vi "xml generate for SFP+_VNA.vi"(0 "input_array_SDD11_Max":string[](array[string]), 1 "input_array_SDD21":string[](array[string]), 2 "路径":path=path "D:/wmgxml.xml", 3 "input_str_label":string, 4 "input_str_CustomerPN":string, 5 "input_array_SCC11_Max":string[](array[string]), 6 "FilePath":string, 7 "input_array_ILD_Max":string[](array[string]), 8 "FileVer":string, 9 "input_array_TDD11":string[](array[string]), 11 "input_array_TDD22":string[](array[string]), 12 "input_array_Next":string[](array[string]), 13 "input_array_time":string[](array[string]), 14 "input_array_impSpec":string[](array[string])) -> ()   [LabVIEW 2011]
panel:
  out "TDD":string
  out "NEXT":string
  out "SCC11":string
  out "SCD21-SDD21":string
  out "ILD":string
  out "SDD11":string
  out "SDD21":string
  in  "input_test_results":bool[](array[boolean])
  out "midVar_time":string[](array[string])
  in  "midVar_state":string
  in  "input_str_product":string
  out "midVar_Content":string
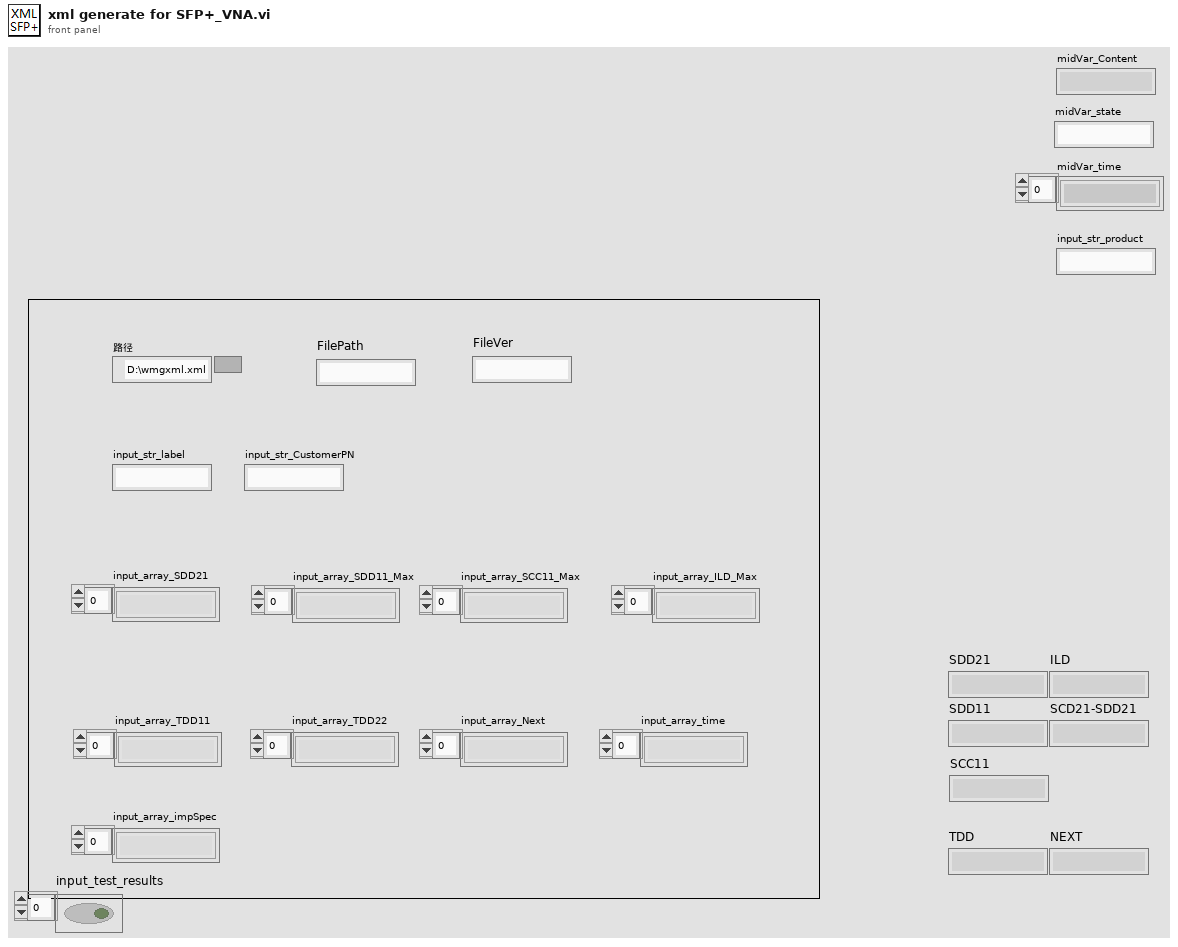
[diagram p1: front panel]
types:
  T1 = enum16{"open", "replace", "create", "open or create", "replace or create", "replace or create with confirmation"}
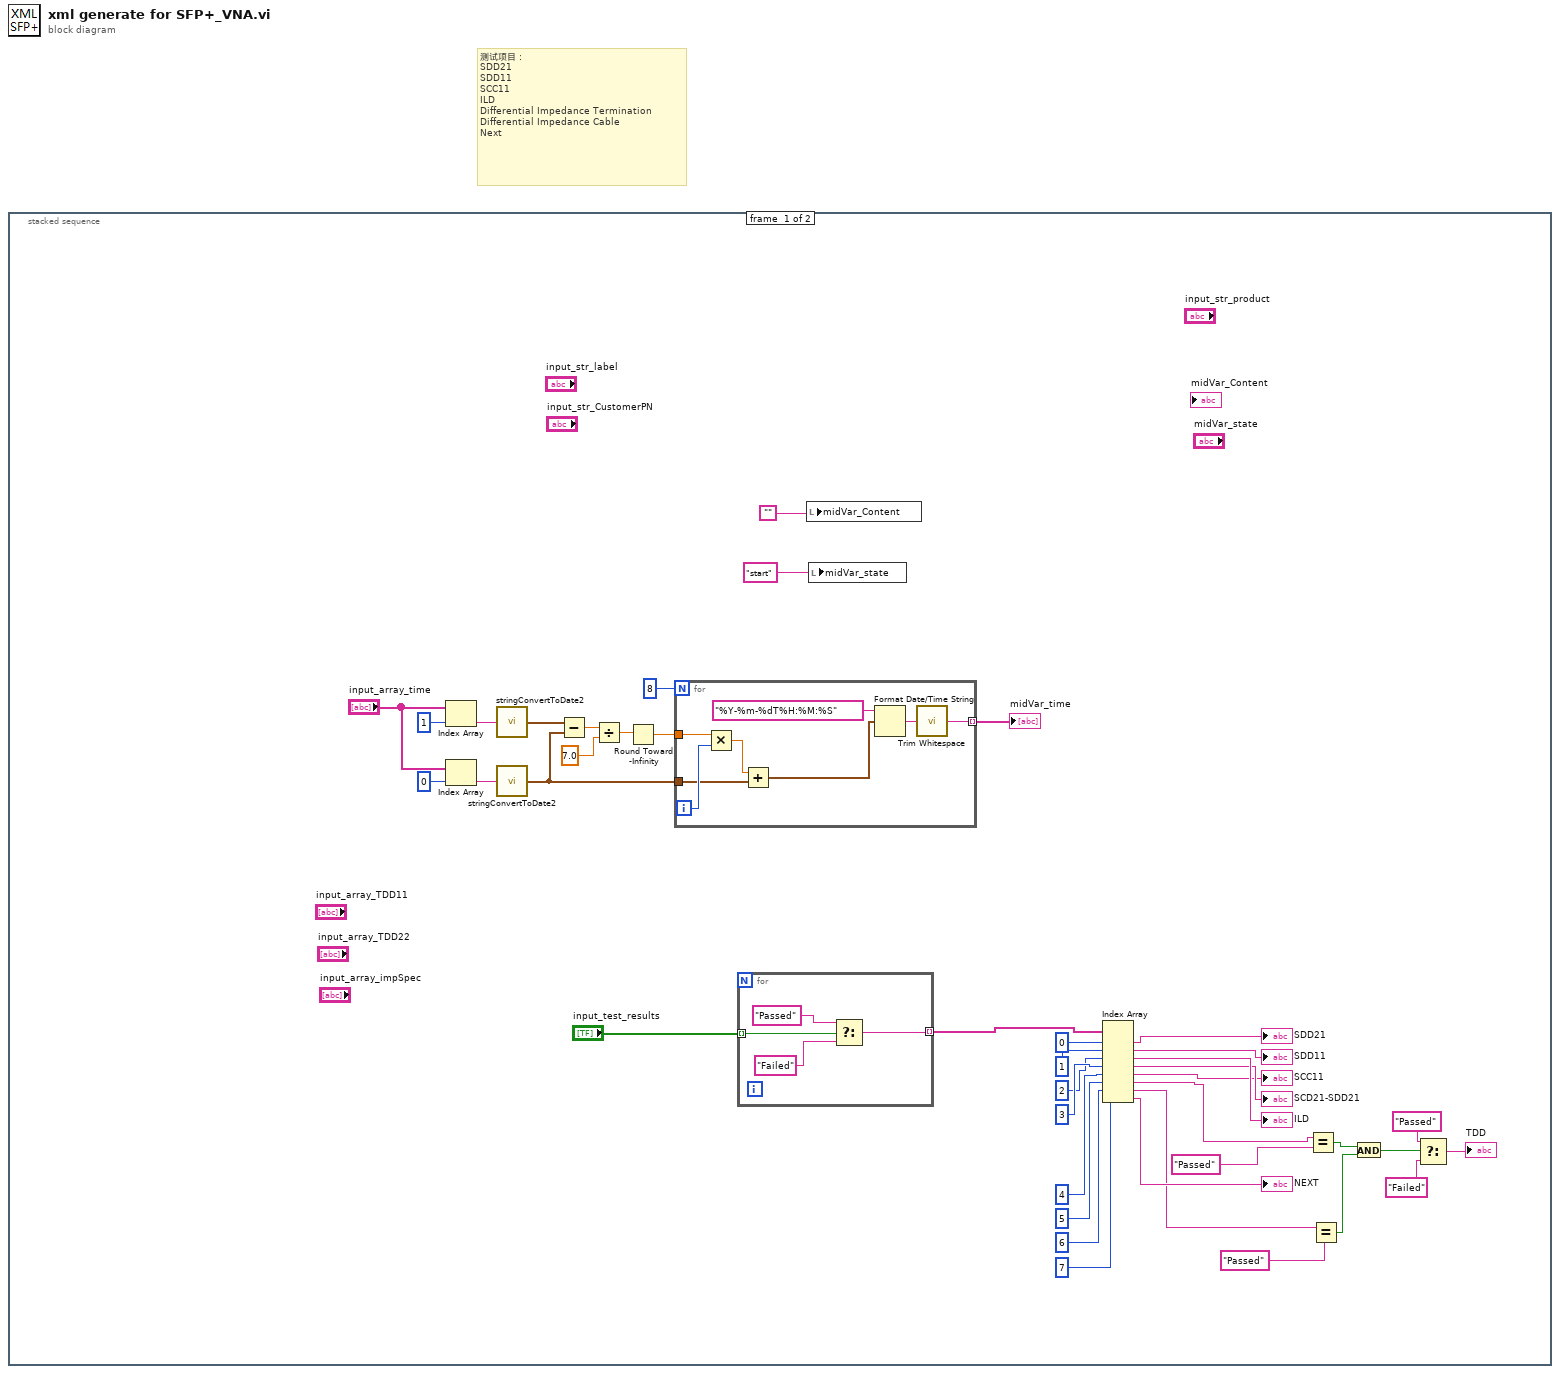
[diagram p0: block diagram]
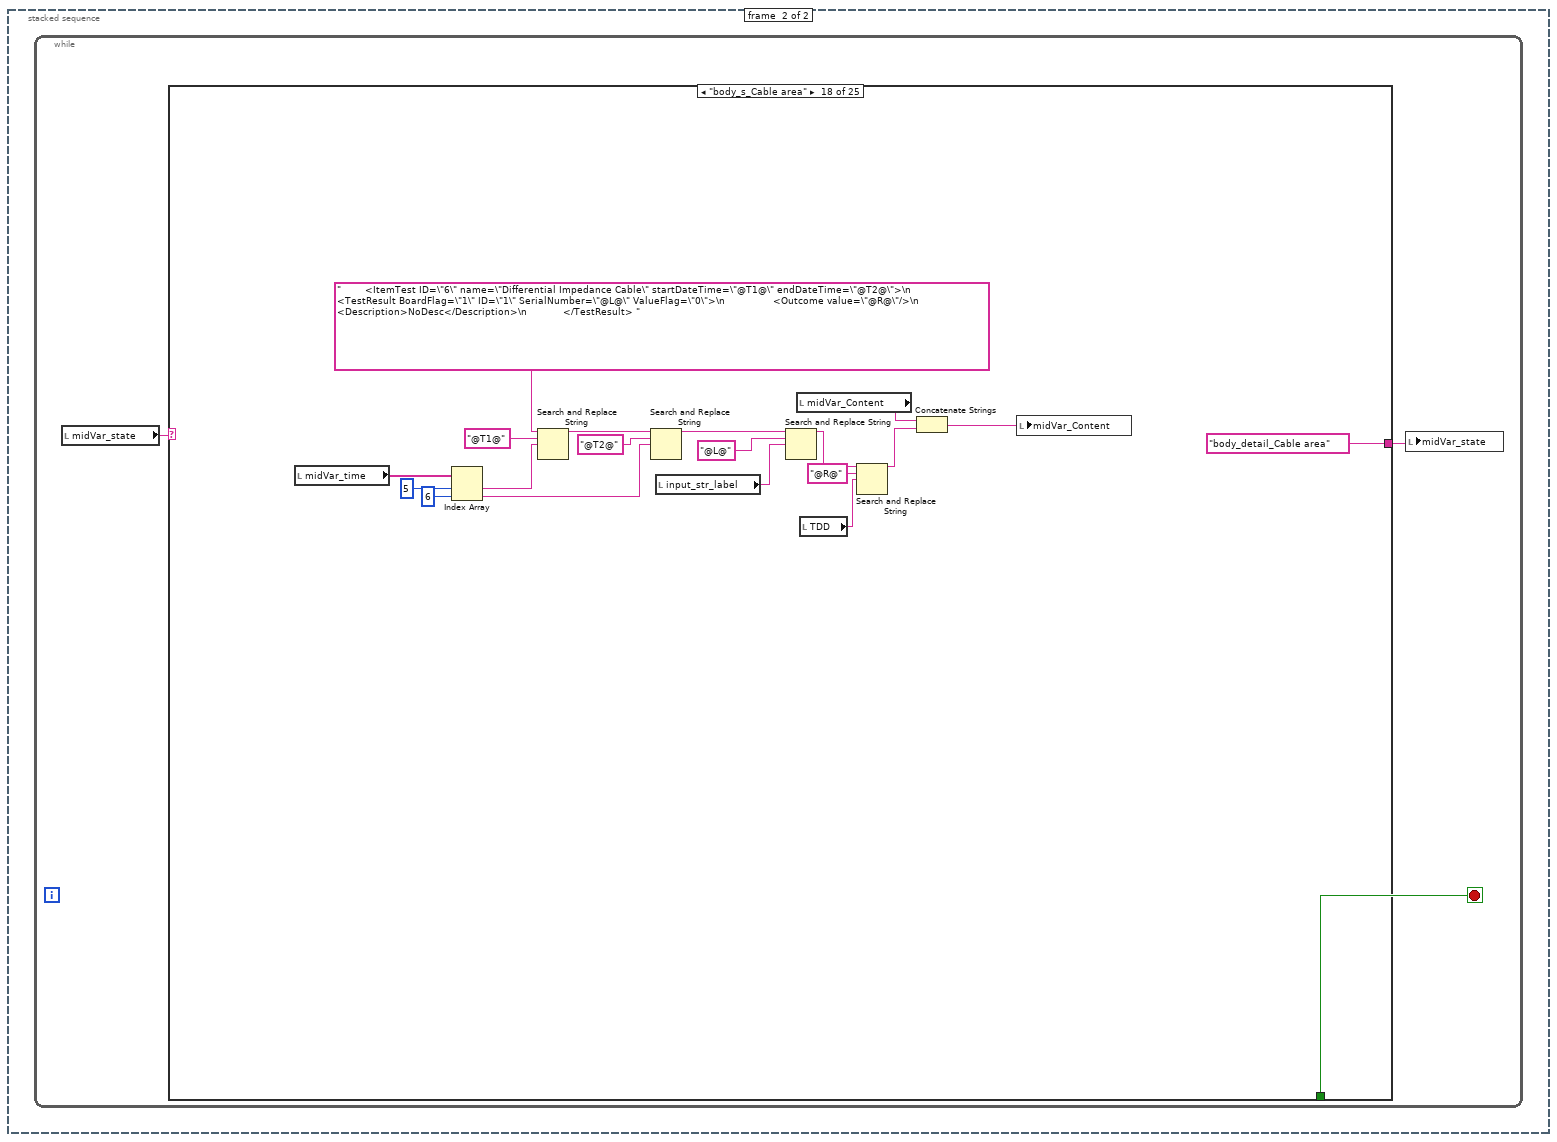
[diagram p2: hidden frame]
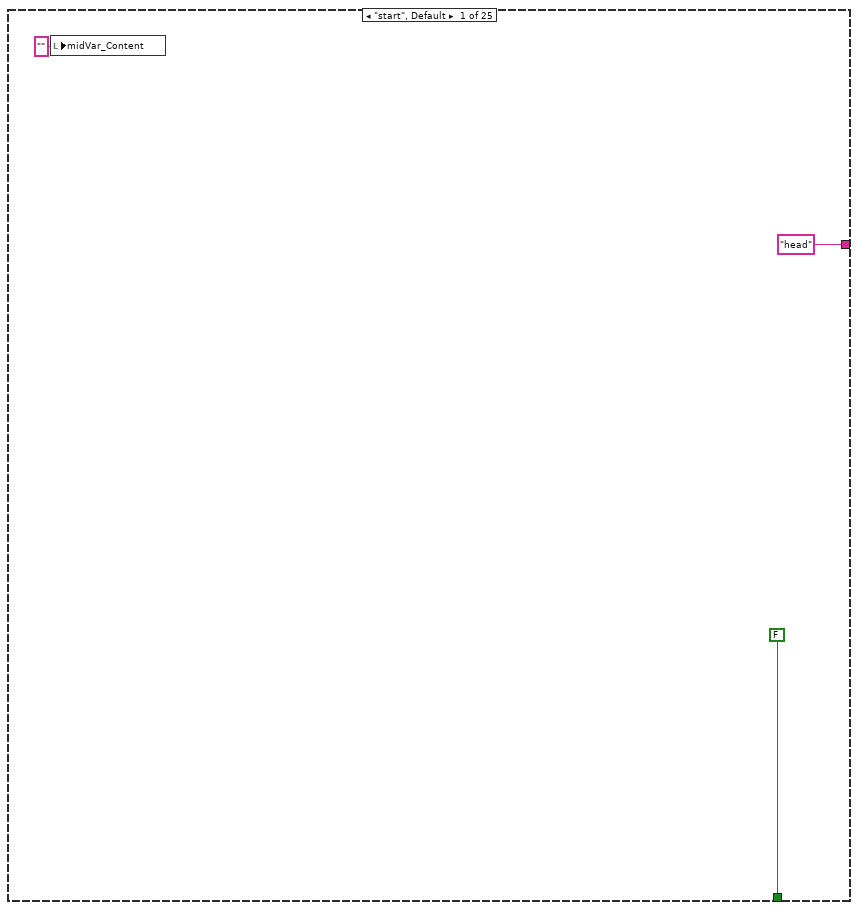
[diagram p3: hidden frame]
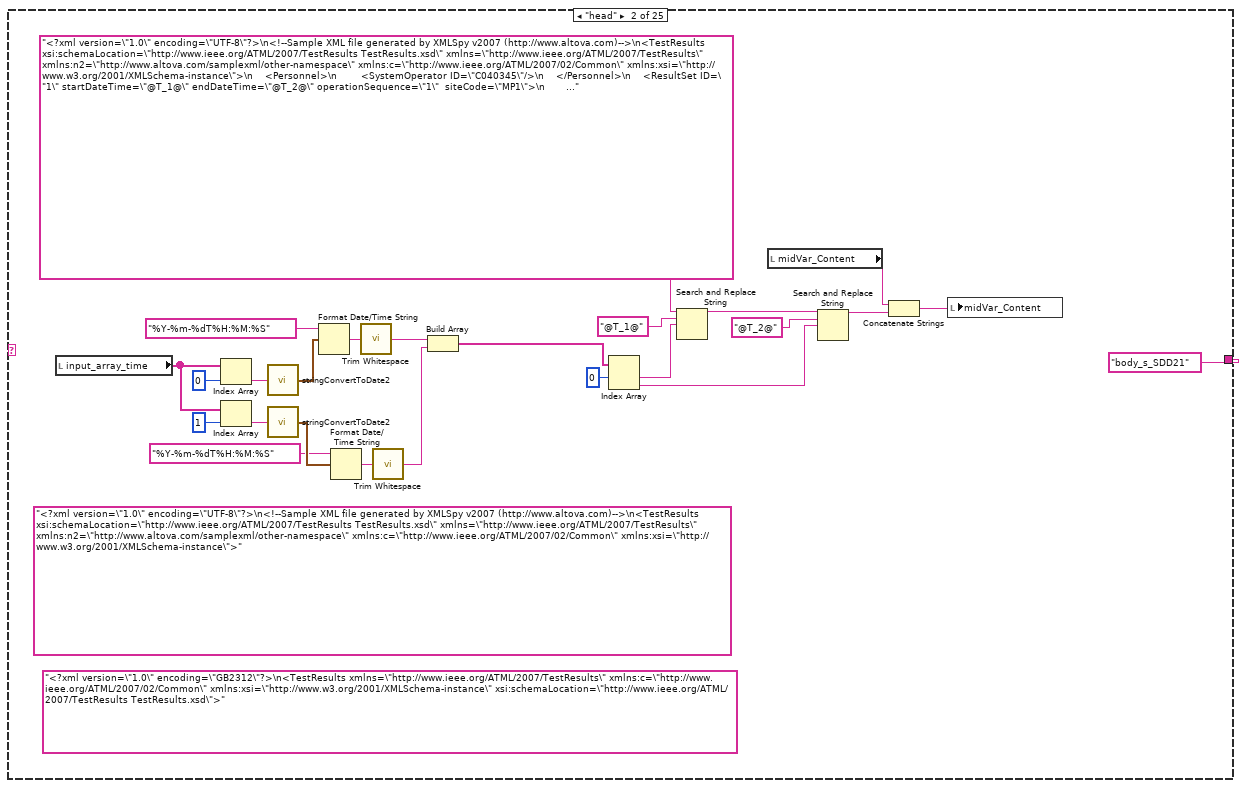
[diagram p4: hidden frame]
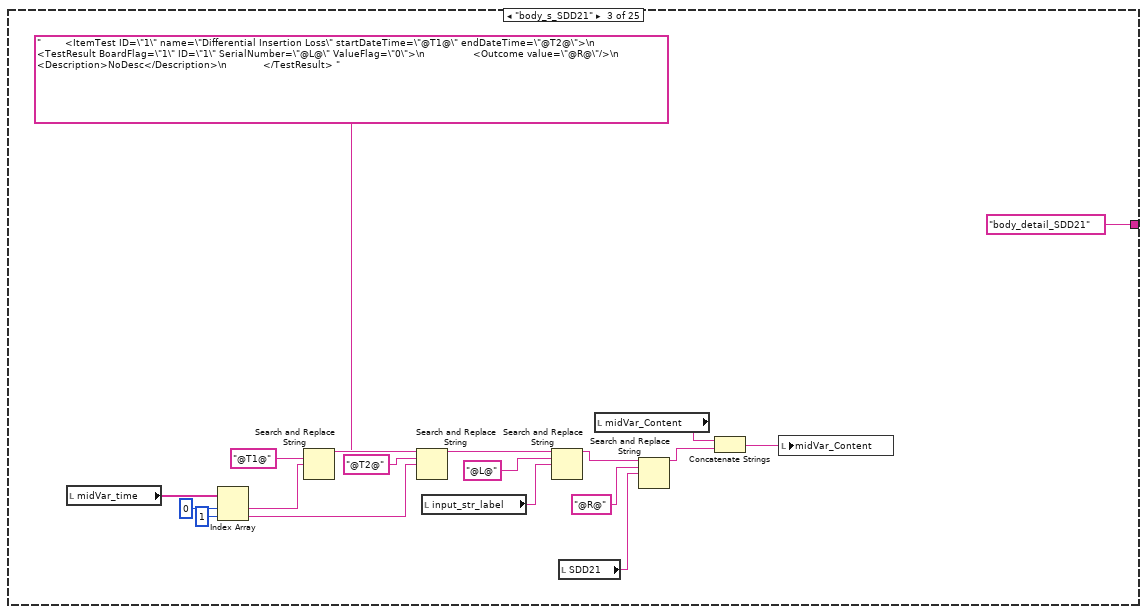
[diagram p5: hidden frame]
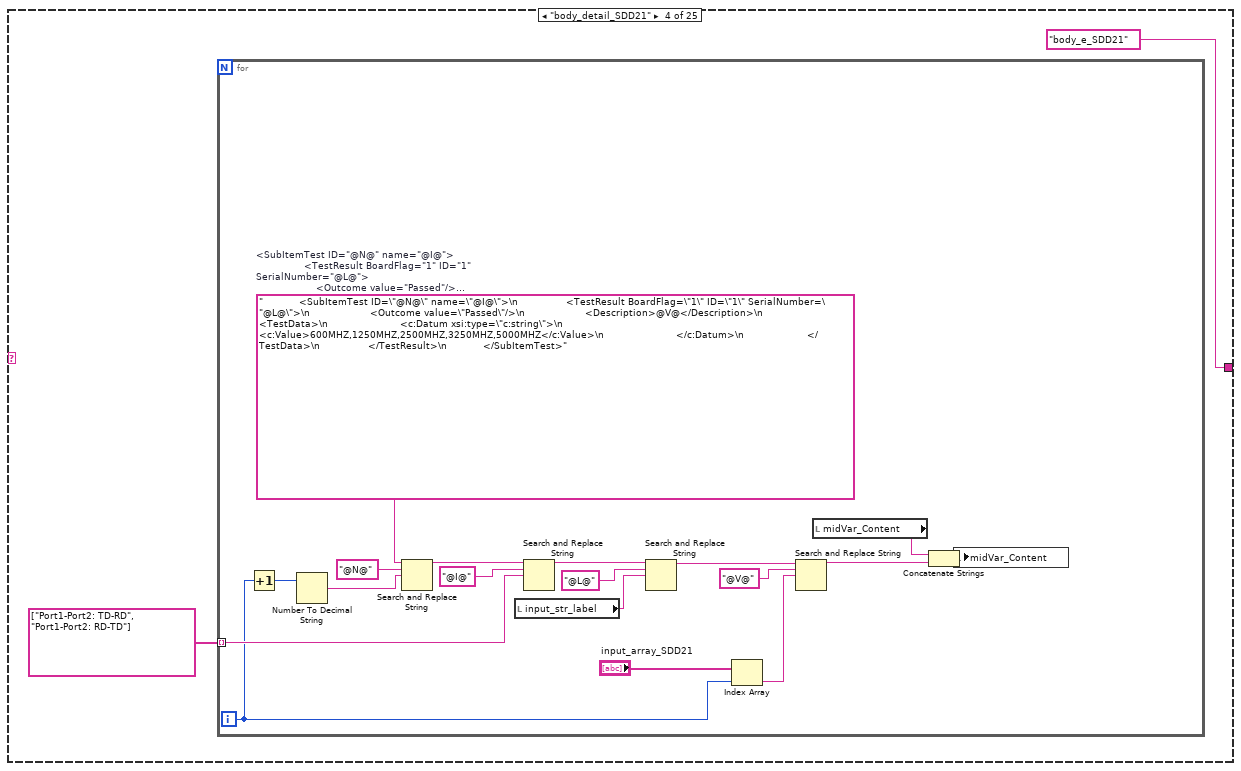
[diagram p6: hidden frame]
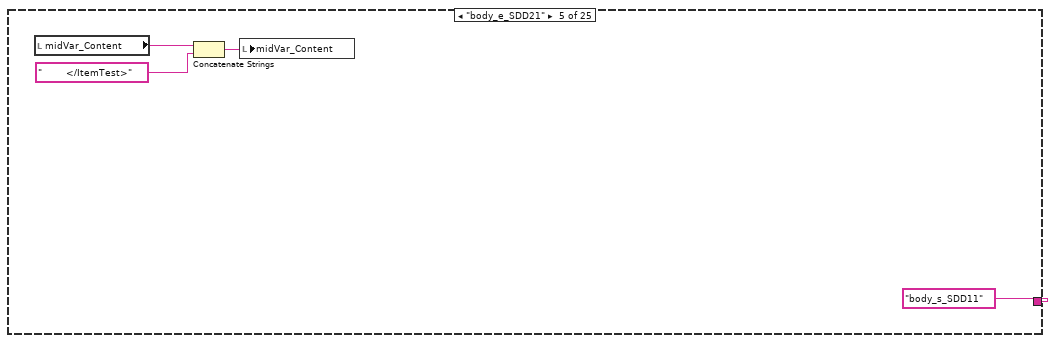
[diagram p7: hidden frame]
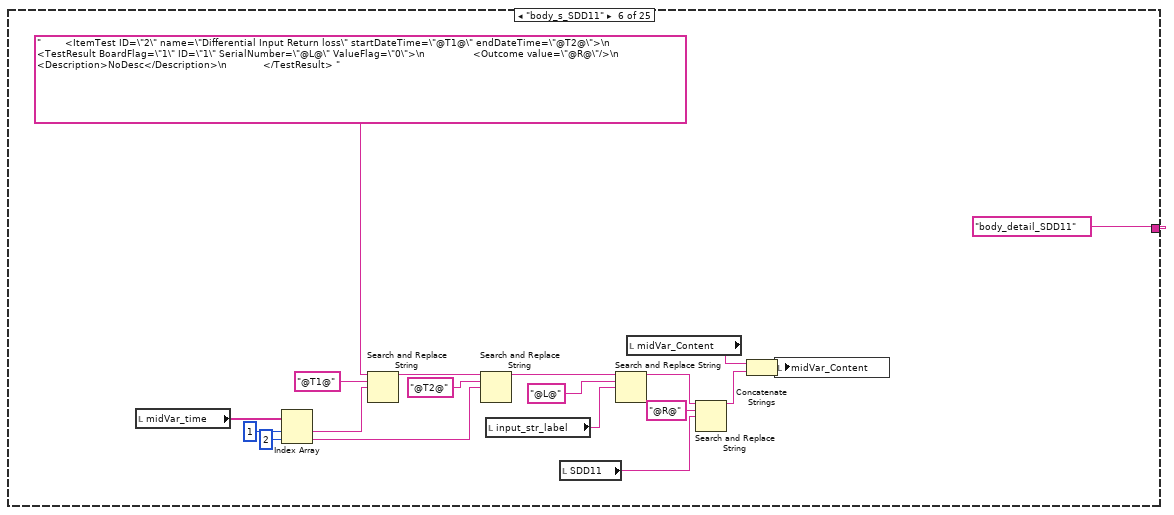
[diagram p8: hidden frame]
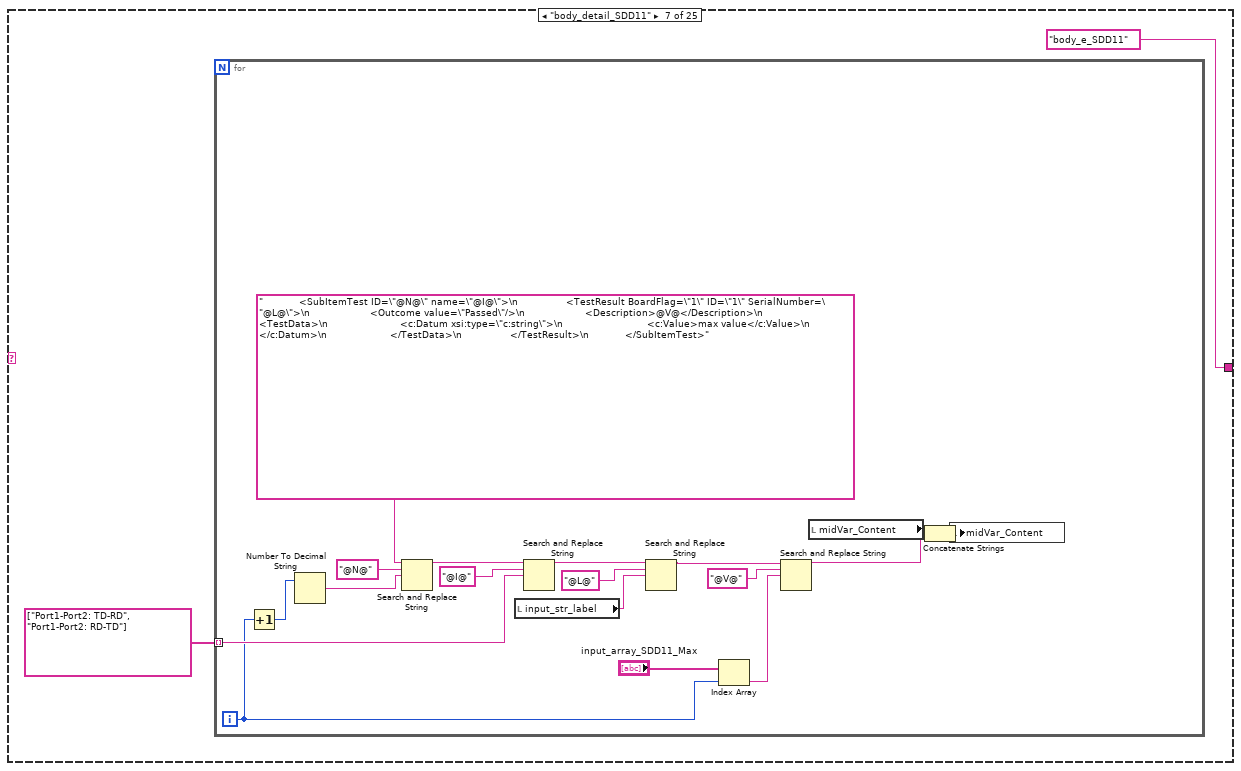
[diagram p9: hidden frame]
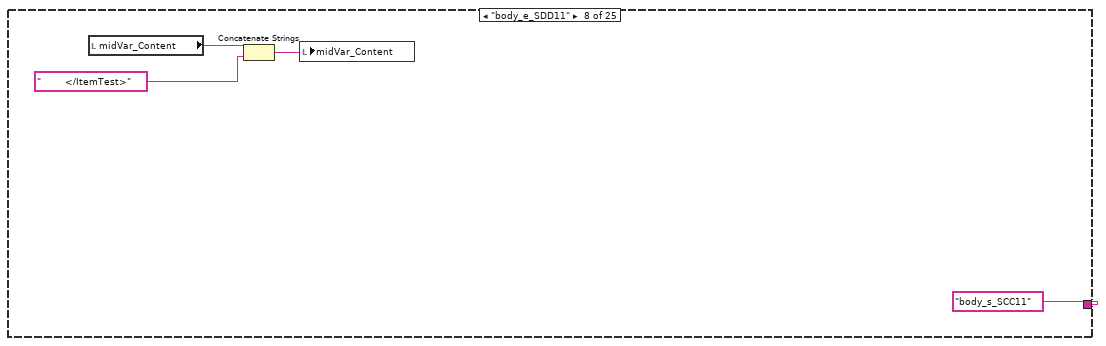
[diagram p10: hidden frame]
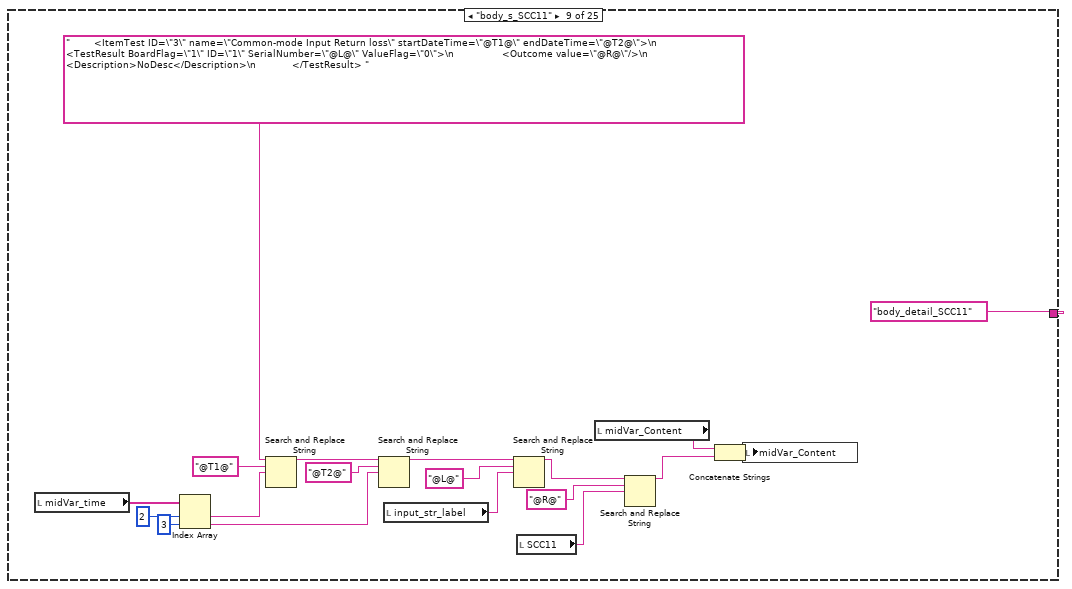
[diagram p11: hidden frame]
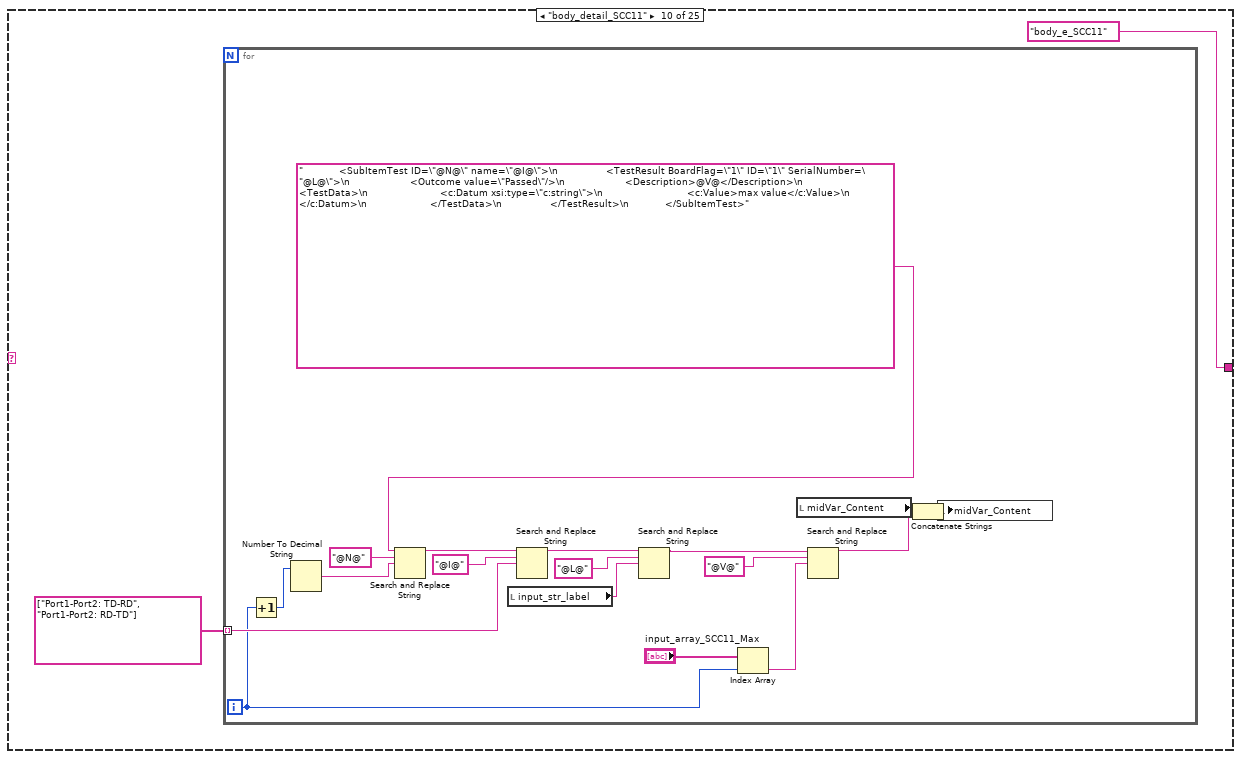
[diagram p12: hidden frame]
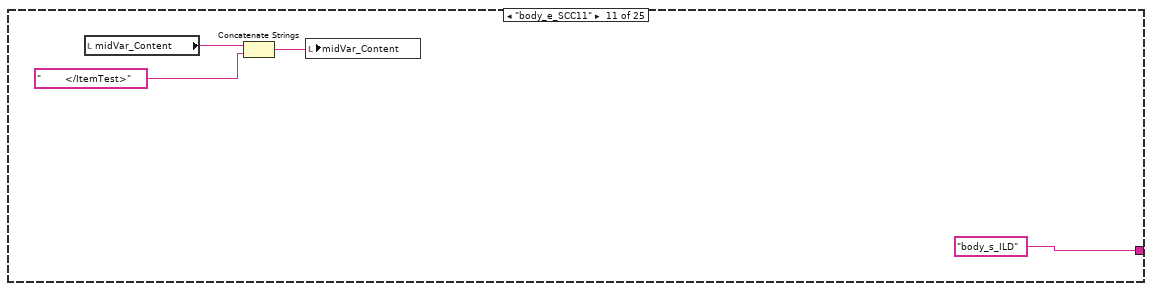
[diagram p13: hidden frame]
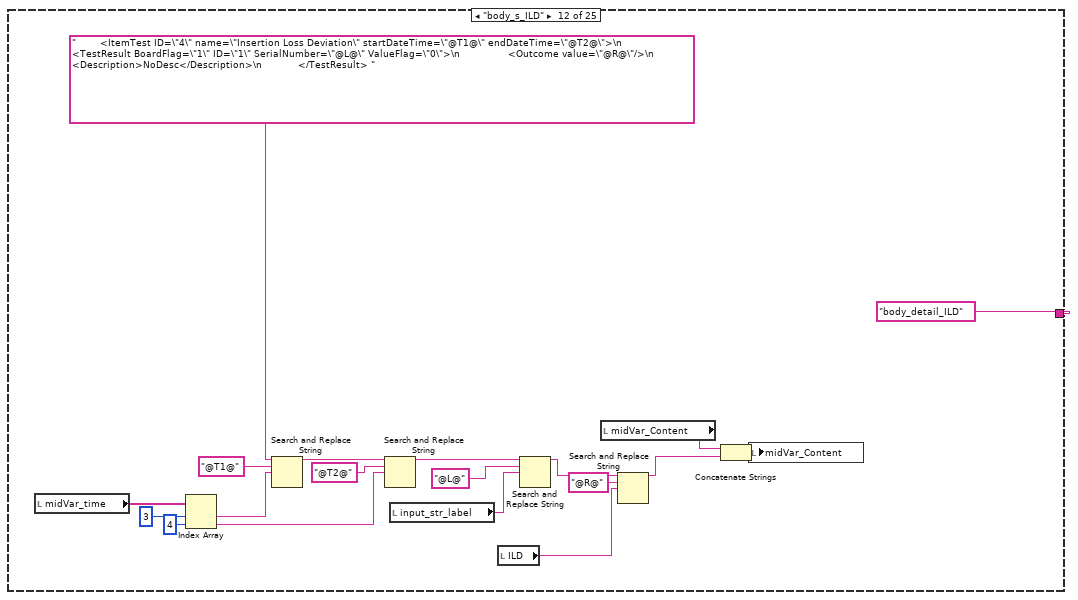
[diagram p14: hidden frame]
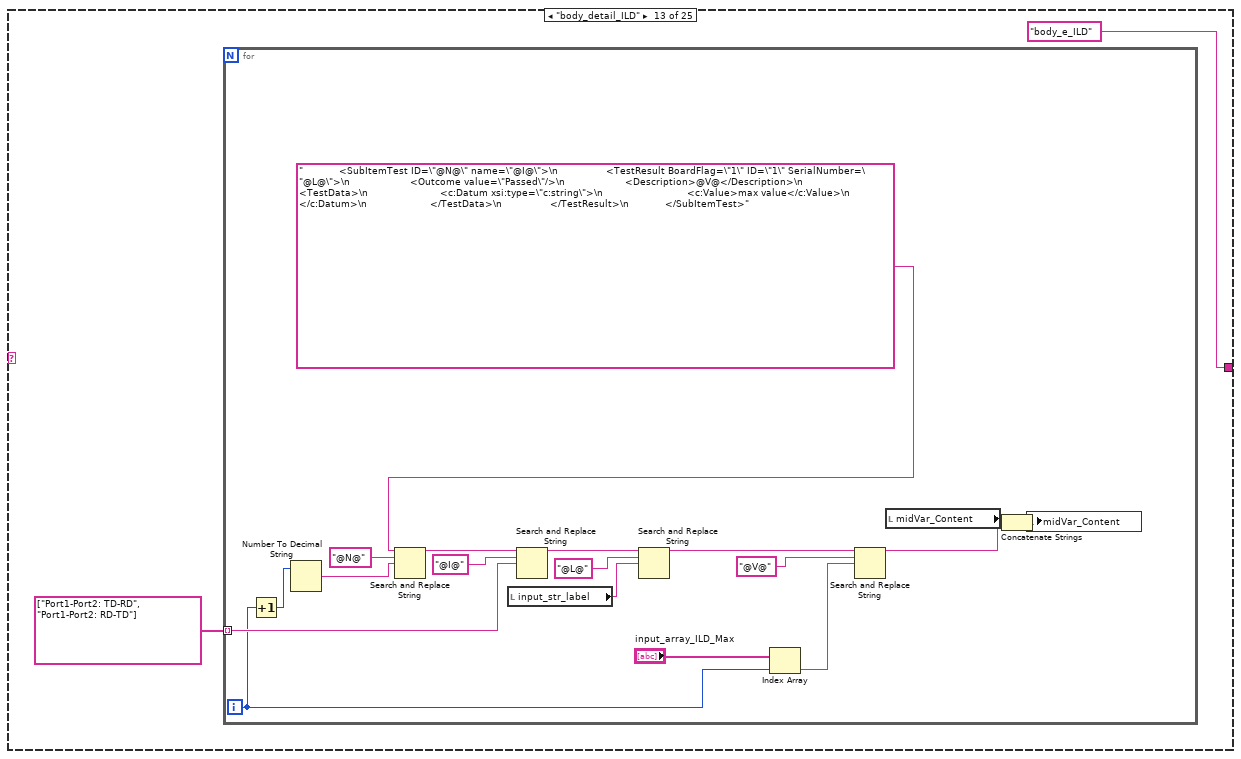
[diagram p15: hidden frame]
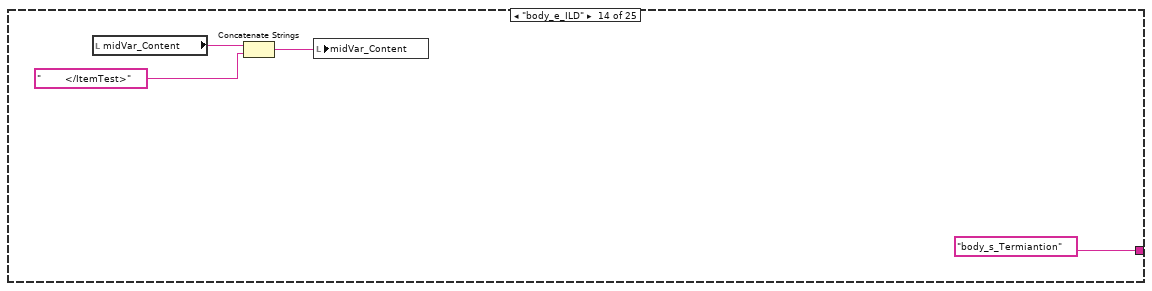
[diagram p16: hidden frame]
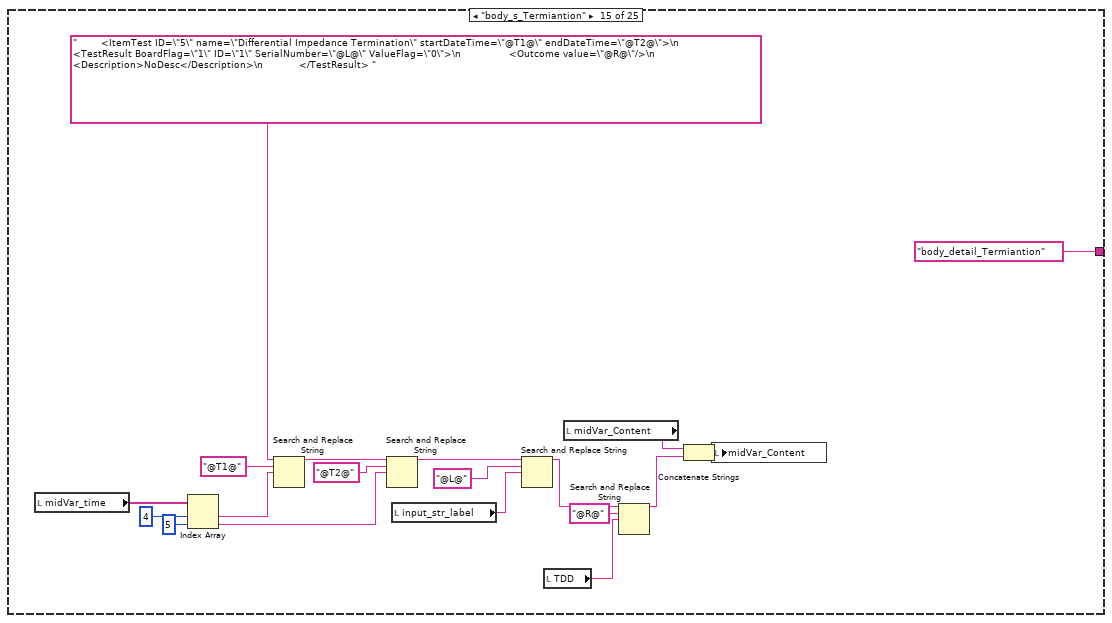
[diagram p17: hidden frame]
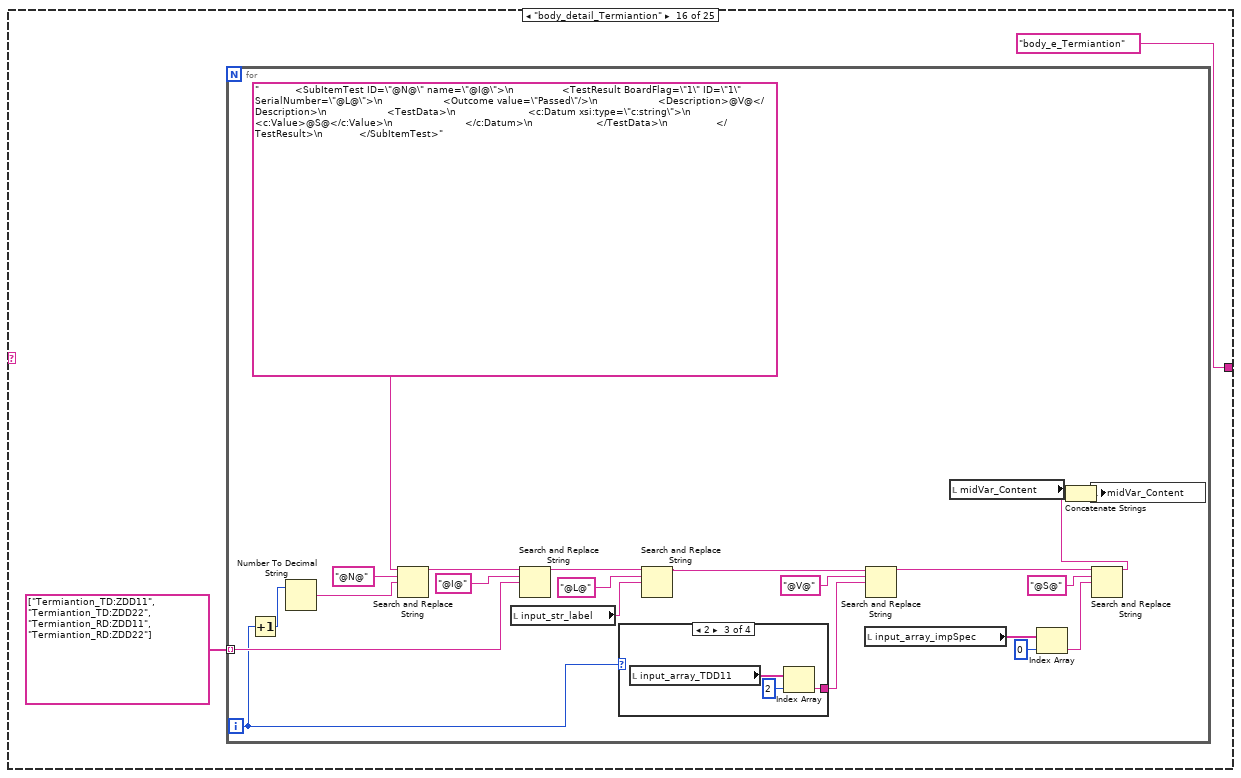
[diagram p18: hidden frame]
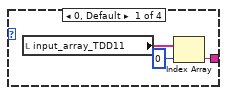
[diagram p19: hidden frame]
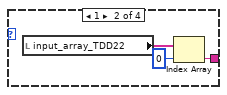
[diagram p20: hidden frame]
diagram:
  # "测试项目：\nSDD21\nSDD11\nSCC11\nILD\nDifferential Impedance Termination\nDifferential Impedance Cable\nNext"
  n1 = stacked-sequence {
    frame #0 {
      n2 = Index Array(array="input_array_time", index=1 ("索引")) -> (element=w30:string)
      n3 = Index Array(array="input_array_time", index=0 ("索引")) -> (element=w31:string)
      n4 = call "stringConvertToDate2.vi"("input_str_yymmdd"=w30) -> ("show_date"=w32:timestamp)
      n5 = call "stringConvertToDate2.vi"("input_str_yymmdd"=w31) -> ("show_date"=w38:timestamp)
      n6 = Subtract(x=w32, y=w38) -> (x-y=w33:dbl)
      n7 = Divide(x=w33, y=7.0) -> (x/y=w35:dbl)
      n8 = Round Toward -Infinity(1:w35) -> (0:w37:dbl)
      n9 = for {
        N: 8 -> [_]
        tunnel: w37 -> [w53]
        tunnel: w38 -> [w51]
        tunnel: [w46] -> w39 mode=indexing
        i -> [w52]
        n10 = Multiply(x=w53, y=w52) -> (x*y=w50:dbl)
        n11 = Add(x=w50, y=w51) -> (x+y=w47:timestamp)
        n12 = Format Date/Time String(time format string (%c)="%Y-%m-%dT%H:%M:%S" ("时间格式字符串(%c)"), seconds (now)=w47) -> (date/time string=w48:string)  [unwired: 1 in]
        n13 = call <vilib>:"Trim Whitespace.vi"("string"=w48) -> ("trimmed string"=w46:string)  [unwired: 1 in]
      }
      "midVar_time" <- w39
      n14 = for {
        tunnel: "input_test_results" -> [w45] mode=indexing
        tunnel: [w42] -> w25 mode=indexing
        n15 = Select(t="Passed", s=w45, f="Failed") -> (s? t:f=w42:string)
      }
      n16 = local write "midVar_Content"("") -> ()
      n17 = local write "midVar_state"("start" ("state")) -> ()
      n18 = Index Array(array=w25, index #1=0 ("索引"), index #2=1 ("索引"), index #3=2 ("索引"), index #4=3 ("索引"), index #5=4 ("索引"), index #6=5 ("索引"), index #7=6 ("索引"), index #8=7 ("索引")) -> (element #1=→"SDD21":string, element #2=→"SDD11":string, element #3=→"ILD":string, element #4=→"SCD21-SDD21":string, element #5=→"SCC11":string, element #6=w11:string, element #7=w9:string, element #8=→"NEXT":string)
      n19 = Equal?(x=w11, y="Passed") -> (x = y?=w7:bool)
      n20 = Equal?(x=w9, y="Passed") -> (x = y?=w6:bool)
      n21 = And(x=w7, y=w6) -> (x .and. y?=w5:bool)
      n22 = Select(t="Passed", s=w5, f="Failed") -> (s? t:f=→"TDD":string)
    }
    frame #1 {
      n23 = while {
        stop <- w54 stop-if-true
        n24 = local read "midVar_state"() -> (w56:string)
        n25 = case shown="\"body_s_Cable area\"" w56 {
          tunnel: ["head" ("state") "body_s_SDD21" ("state") "body_detail_SDD21" "body_e_SDD21" "body_s_SDD11" "body_detail_SDD11" "body_e_SDD11" "body_s_SCC11" "body_detail_SCC11" "body_e_SCC11" "body_s_ILD" "body_detail_ILD" "body_e_ILD" "body_s_Termiantion" "body_detail_Termiantion" "body_e_Termiantion" "body_s_Cable area" "body_detail_Cable area" "body_e_Cable area" "body_s_Next" "body_detail_Next" "body_e_Next" "tail" "end" ("state") "start" ("state")] -> w55
          tunnel: [FALSE _ _ _ _ _ _ _ _ _ _ _ _ _ _ _ _ _ _ _ _ _ _ _ TRUE] -> w54
          frame "start", Default {
            n26 = local write "midVar_Content"("" ("字符串")) -> ()
          }
          frame "head" {
            (unwired) "<?xml version=\"1.0\" encoding=\"GB2312\"?>\n<TestResults xmlns=\"http://www.ieee.org/ATML/2007/TestResults\" xmlns:c=\"http://www.ieee.org/ATML/2007/02/Common\" xmlns:xsi=\"http://www.w3.org/2001/XMLSchema-instance\" xsi:schemaLocation=\"http://www.ieee.org/ATML/2007/TestResults TestResults.xsd\">"
            (unwired) "<?xml version=\"1.0\" encoding=\"UTF-8\"?>\n<!--Sample XML file generated by XMLSpy v2007 (http://www.altova.com)-->\n<TestResults xsi:schemaLocation=\"http://www.ieee.org/ATML/2007/TestResults TestResults.xsd\" xmlns=\"http://www.ieee.org/ATML/2007/TestResults\" xmlns:n2=\"http://www.altova.com/samplexml/other-namespace\" xmlns:c=\"http://www.ieee.org/ATML/2007/02/Common\" xmlns:xsi=\"http://www.w3.org/2001/XMLSchema-instance\">"
            n27 = local read "input_array_time"() -> (w69:string[])
            n28 = Index Array(array=w69, index=0 ("索引")) -> (element=w68:string)
            n29 = Index Array(array=w69, index=1 ("索引")) -> (element=w67:string)
            n30 = call "stringConvertToDate2.vi"("input_str_yymmdd"=w68) -> ("show_date"=w65:timestamp)
            n31 = call "stringConvertToDate2.vi"("input_str_yymmdd"=w67) -> ("show_date"=w64:timestamp)
            n32 = Format Date/Time String(time format string (%c)="%Y-%m-%dT%H:%M:%S" ("时间格式字符串(%c)"), seconds (now)=w65) -> (date/time string=w72:string)  [unwired: 1 in]
            n33 = Format Date/Time String(time format string (%c)="%Y-%m-%dT%H:%M:%S" ("时间格式字符串(%c)"), seconds (now)=w64) -> (date/time string=w66:string)  [unwired: 1 in]
            n34 = call <vilib>:"Trim Whitespace.vi"("string"=w72) -> ("trimmed string"=w62:string)  [unwired: 1 in]
            n35 = call <vilib>:"Trim Whitespace.vi"("string"=w66) -> ("trimmed string"=w61:string)  [unwired: 1 in]
            n36 = Build Array(w62, w61) -> (w60:string[])
            n37 = Index Array(array=w60, index #1=0 ("索引")) -> (element #1=w82:string, element #2=w79:string)  [unwired: 1 in]
            n38 = Search and Replace String(input string="<?xml version=\"1.0\" encoding=\"UTF-8\"?>\n<!--Sample XML file generated by XMLSpy v2007 (http://www.altova.com)-->\n<TestResults xsi:schemaLocation=\"http://www.ieee.org/ATML/2007/TestResults TestResults.xsd\" xmlns=\"http://www.ieee.org/ATML/2007/TestResults\" xmlns:n2=\"http://www.altova.com/samplexml/other-namespace\" xmlns:c=\"http://www.ieee.org/ATML/2007/02/Common\" xmlns:xsi=\"http://www.w3.org/2001/XMLSchema-instance\">\n    <Personnel>\n        <SystemOperator ID=\"C040345\"/>\n    </Personnel>\n    <ResultSet ID=\"1\" startDateTime=\"@T_1@\" endDateTime=\"@T_2@\" operationSequence=\"1\"  siteCode=\"MP1\">\n        <Description>CMZ00A2R</Description>\n        <TestResult BoardFlag=\"1\" ID=\"1\">\n            <Outcome value=\"Passed\"/>\n        </TestResult>", search string="@T_1@" ("搜索字符串"), replace string=w82) -> (result string=w81:string)  [unwired: 5 in, 3 out]
            n39 = local read "midVar_Content"() -> (w77:string)
            n40 = Search and Replace String(input string=w81, search string="@T_2@" ("搜索字符串"), replace string=w79) -> (result string=w74:string)  [unwired: 5 in, 3 out]
            n41 = Concatenate Strings(w77, w74) -> (w76:string)
            n42 = local write "midVar_Content"(w76) -> ()
          }
          frame "body_s_SDD21" {
            n43 = local read "midVar_time"() -> (w90:string[])
            n44 = Index Array(array=w90, index #1=0 ("索引"), index #2=1 ("索引")) -> (element #1=w101:string, element #2=w98:string)
            n45 = Search and Replace String(input string="        <ItemTest ID=\"1\" name=\"Differential Insertion Loss\" startDateTime=\"@T1@\" endDateTime=\"@T2@\">\n            <TestResult BoardFlag=\"1\" ID=\"1\" SerialNumber=\"@L@\" ValueFlag=\"0\">\n                <Outcome value=\"@R@\"/>\n                <Description>NoDesc</Description>\n            </TestResult> ", search string="@T1@" ("搜索字符串"), replace string=w101) -> (result string=w100:string)  [unwired: 5 in, 3 out]
            n46 = Search and Replace String(input string=w100, search string="@T2@" ("搜索字符串"), replace string=w98) -> (result string=w93:string)  [unwired: 5 in, 3 out]
            n47 = local read "input_str_label"() -> (w92:string)
            n48 = Search and Replace String(input string=w93, search string="@L@" ("搜索字符串"), replace string=w92) -> (result string=w88:string)  [unwired: 5 in, 3 out]
            n49 = local read "SDD21"() -> (w85:string)
            n50 = local read "midVar_Content"() -> (w97:string)
            n51 = Search and Replace String(input string=w88, search string="@R@" ("搜索字符串"), replace string=w85) -> (result string=w87:string)  [unwired: 5 in, 3 out]
            n52 = Concatenate Strings(w97, w87) -> (w96:string)
            n53 = local write "midVar_Content"(w96) -> ()
          }
          frame "body_detail_SDD21" {
            n54 = for {
              tunnel: string[] ["Port1-Port2: TD-RD", "Port1-Port2: RD-TD"] -> [w118] mode=indexing
              i -> [w108]
              w123 = "            <SubItemTest ID=\"@N@\" name=\"@I@\">\n                <TestResult BoardFlag=\"1\" ID=\"1\" SerialNumber=\"@L@\">\n                    <Outcome value=\"Passed\"/>\n                    <Description>@V@</Description>\n                    <TestData>\n                        <c:Datum xsi:type=\"c:string\">\n                            <c:Value>600MHZ,1250MHZ,2500MHZ,3250MHZ,5000MHZ</c:Value>\n                        </c:Datum>\n                     </TestData>\n                </TestResult>\n            </SubItemTest>"  # <SubItemTest ID="@N@" name="@I@">                 <TestResult BoardFlag="1" ID="1" SerialNumber="@L@">                     <Outcome value="Passed"/>                     <Description>@V@</Description>                     <TestData>                         <c:Datum xsi:type="c:string">                             <c:Value>600MHZ,1250MHZ,2500MHZ,3250MHZ,5000MHZ</c:Value>                         </c:Datum>                      </TestData>                 </TestResult>             </SubItemTest>
              n55 = Increment(x=w108) -> (x+1=w110:i32)
              n56 = Number To Decimal String(number=w110) -> (decimal integer string=w121:string)  [unwired: 1 in]
              n57 = Search and Replace String(input string=w123, search string="@N@" ("搜索字符串"), replace string=w121) -> (result string=w120:string)  [unwired: 5 in, 3 out]
              n58 = local read "input_str_label"() -> (w115:string)
              n59 = Search and Replace String(input string=w120, search string="@I@" ("搜索字符串"), replace string=w118) -> (result string=w117:string)  [unwired: 5 in, 3 out]
              n60 = Search and Replace String(input string=w117, search string="@L@" ("搜索字符串"), replace string=w115) -> (result string=w109:string)  [unwired: 5 in, 3 out]
              n61 = Index Array(array="input_array_SDD21", index=w108) -> (element=w112:string)
              n62 = Search and Replace String(input string=w109, search string="@V@" ("搜索字符串"), replace string=w112) -> (result string=w106:string)  [unwired: 5 in, 3 out]
              n63 = local read "midVar_Content"() -> (w114:string)
              n64 = Concatenate Strings(w114, w106) -> (w111:string)
              n65 = local write "midVar_Content"(w111) -> ()
            }
          }
          frame "body_e_SDD21" {
            n66 = local read "midVar_Content"() -> (w127:string)
            n67 = Concatenate Strings(w127, "        </ItemTest>") -> (w126:string)
            n68 = local write "midVar_Content"(w126) -> ()
          }
          frame "body_s_SDD11" {
            n69 = local read "midVar_time"() -> (w133:string[])
            n70 = Index Array(array=w133, index #1=1 ("索引"), index #2=2 ("索引")) -> (element #1=w144:string, element #2=w141:string)
            n71 = Search and Replace String(input string="        <ItemTest ID=\"2\" name=\"Differential Input Return loss\" startDateTime=\"@T1@\" endDateTime=\"@T2@\">\n            <TestResult BoardFlag=\"1\" ID=\"1\" SerialNumber=\"@L@\" ValueFlag=\"0\">\n                <Outcome value=\"@R@\"/>\n                <Description>NoDesc</Description>\n            </TestResult> ", search string="@T1@" ("搜索字符串"), replace string=w144) -> (result string=w143:string)  [unwired: 5 in, 3 out]
            n72 = Search and Replace String(input string=w143, search string="@T2@" ("搜索字符串"), replace string=w141) -> (result string=w136:string)  [unwired: 5 in, 3 out]
            n73 = local read "input_str_label"() -> (w135:string)
            n74 = local read "SDD11"() -> (w128:string)
            n75 = Search and Replace String(input string=w136, search string="@L@" ("搜索字符串"), replace string=w135) -> (result string=w131:string)  [unwired: 5 in, 3 out]
            n76 = local read "midVar_Content"() -> (w140:string)
            n77 = Search and Replace String(input string=w131, search string="@R@" ("搜索字符串"), replace string=w128) -> (result string=w130:string)  [unwired: 5 in, 3 out]
            n78 = Concatenate Strings(w140, w130) -> (w139:string)
            n79 = local write "midVar_Content"(w139) -> ()
          }
          frame "body_detail_SDD11" {
            n80 = for {
              tunnel: string[] ["Port1-Port2: TD-RD", "Port1-Port2: RD-TD"] -> [w161] mode=indexing
              i -> [w151]
              n81 = Increment(x=w151) -> (x+1=w153:i32)
              n82 = Number To Decimal String(number=w153) -> (decimal integer string=w164:string)  [unwired: 1 in]
              n83 = Search and Replace String(input string="            <SubItemTest ID=\"@N@\" name=\"@I@\">\n                <TestResult BoardFlag=\"1\" ID=\"1\" SerialNumber=\"@L@\">\n                    <Outcome value=\"Passed\"/>\n                    <Description>@V@</Description>\n                    <TestData>\n                        <c:Datum xsi:type=\"c:string\">\n                            <c:Value>max value</c:Value>\n                        </c:Datum>\n                     </TestData>\n                </TestResult>\n            </SubItemTest>", search string="@N@" ("搜索字符串"), replace string=w164) -> (result string=w163:string)  [unwired: 5 in, 3 out]
              n84 = local read "input_str_label"() -> (w158:string)
              n85 = Search and Replace String(input string=w163, search string="@I@" ("搜索字符串"), replace string=w161) -> (result string=w160:string)  [unwired: 5 in, 3 out]
              n86 = Search and Replace String(input string=w160, search string="@L@" ("搜索字符串"), replace string=w158) -> (result string=w152:string)  [unwired: 5 in, 3 out]
              n87 = Index Array(array="input_array_SDD11_Max", index=w151) -> (element=w155:string)
              n88 = Search and Replace String(input string=w152, search string="@V@" ("搜索字符串"), replace string=w155) -> (result string=w149:string)  [unwired: 5 in, 3 out]
              n89 = local read "midVar_Content"() -> (w157:string)
              n90 = Concatenate Strings(w157, w149) -> (w154:string)
              n91 = local write "midVar_Content"(w154) -> ()
            }
          }
          frame "body_e_SDD11" {
            n92 = local read "midVar_Content"() -> (w170:string)
            n93 = Concatenate Strings(w170, "        </ItemTest>") -> (w169:string)
            n94 = local write "midVar_Content"(w169) -> ()
          }
          frame "body_s_SCC11" {
            n95 = local read "midVar_time"() -> (w176:string[])
            n96 = Index Array(array=w176, index #1=2 ("索引"), index #2=3 ("索引")) -> (element #1=w187:string, element #2=w184:string)
            n97 = Search and Replace String(input string="        <ItemTest ID=\"3\" name=\"Common-mode Input Return loss\" startDateTime=\"@T1@\" endDateTime=\"@T2@\">\n            <TestResult BoardFlag=\"1\" ID=\"1\" SerialNumber=\"@L@\" ValueFlag=\"0\">\n                <Outcome value=\"@R@\"/>\n                <Description>NoDesc</Description>\n            </TestResult> ", search string="@T1@" ("搜索字符串"), replace string=w187) -> (result string=w186:string)  [unwired: 5 in, 3 out]
            n98 = Search and Replace String(input string=w186, search string="@T2@" ("搜索字符串"), replace string=w184) -> (result string=w179:string)  [unwired: 5 in, 3 out]
            n99 = local read "input_str_label"() -> (w178:string)
            n100 = Search and Replace String(input string=w179, search string="@L@" ("搜索字符串"), replace string=w178) -> (result string=w174:string)  [unwired: 5 in, 3 out]
            n101 = local read "SCC11"() -> (w171:string)
            n102 = local read "midVar_Content"() -> (w183:string)
            n103 = Search and Replace String(input string=w174, search string="@R@" ("替换字符串(\"\")"), replace string=w171) -> (result string=w173:string)  [unwired: 5 in, 3 out]
            n104 = Concatenate Strings(w183, w173) -> (w182:string)
            n105 = local write "midVar_Content"(w182) -> ()
          }
          frame "body_detail_SCC11" {
            n106 = for {
              tunnel: string[] ["Port1-Port2: TD-RD", "Port1-Port2: RD-TD"] -> [w205] mode=indexing
              i -> [w192]
              n107 = Increment(x=w192) -> (x+1=w197:i32)
              n108 = Number To Decimal String(number=w197) -> (decimal integer string=w208:string)  [unwired: 1 in]
              n109 = Search and Replace String(input string="            <SubItemTest ID=\"@N@\" name=\"@I@\">\n                <TestResult BoardFlag=\"1\" ID=\"1\" SerialNumber=\"@L@\">\n                    <Outcome value=\"Passed\"/>\n                    <Description>@V@</Description>\n                    <TestData>\n                        <c:Datum xsi:type=\"c:string\">\n                            <c:Value>max value</c:Value>\n                        </c:Datum>\n                     </TestData>\n                </TestResult>\n            </SubItemTest>", search string="@N@" ("搜索字符串"), replace string=w208) -> (result string=w207:string)  [unwired: 5 in, 3 out]
              n110 = local read "input_str_label"() -> (w202:string)
              n111 = Search and Replace String(input string=w207, search string="@I@" ("搜索字符串"), replace string=w205) -> (result string=w204:string)  [unwired: 5 in, 3 out]
              n112 = Search and Replace String(input string=w204, search string="@L@" ("搜索字符串"), replace string=w202) -> (result string=w195:string)  [unwired: 5 in, 3 out]
              n113 = Index Array(array="input_array_SCC11_Max", index=w192) -> (element=w199:string)
              n114 = local read "midVar_Content"() -> (w201:string)
              n115 = Search and Replace String(input string=w195, search string="@V@" ("搜索字符串"), replace string=w199) -> (result string=w194:string)  [unwired: 5 in, 3 out]
              n116 = Concatenate Strings(w201, w194) -> (w198:string)
              n117 = local write "midVar_Content"(w198) -> ()
            }
          }
          frame "body_e_SCC11" {
            n118 = local read "midVar_Content"() -> (w213:string)
            n119 = Concatenate Strings(w213, "        </ItemTest>") -> (w212:string)
            n120 = local write "midVar_Content"(w212) -> ()
          }
          frame "body_s_ILD" {
            n121 = local read "midVar_time"() -> (w219:string[])
            n122 = Index Array(array=w219, index #1=3 ("索引"), index #2=4 ("索引")) -> (element #1=w230:string, element #2=w227:string)
            n123 = Search and Replace String(input string="        <ItemTest ID=\"4\" name=\"Insertion Loss Deviation\" startDateTime=\"@T1@\" endDateTime=\"@T2@\">\n            <TestResult BoardFlag=\"1\" ID=\"1\" SerialNumber=\"@L@\" ValueFlag=\"0\">\n                <Outcome value=\"@R@\"/>\n                <Description>NoDesc</Description>\n            </TestResult> ", search string="@T1@" ("搜索字符串"), replace string=w230) -> (result string=w229:string)  [unwired: 5 in, 3 out]
            n124 = Search and Replace String(input string=w229, search string="@T2@" ("搜索字符串"), replace string=w227) -> (result string=w222:string)  [unwired: 5 in, 3 out]
            n125 = local read "input_str_label"() -> (w221:string)
            n126 = local read "ILD"() -> (w214:string)
            n127 = Search and Replace String(input string=w222, search string="@L@" ("搜索字符串"), replace string=w221) -> (result string=w217:string)  [unwired: 5 in, 3 out]
            n128 = local read "midVar_Content"() -> (w226:string)
            n129 = Search and Replace String(input string=w217, search string="@R@" ("搜索字符串"), replace string=w214) -> (result string=w216:string)  [unwired: 5 in, 3 out]
            n130 = Concatenate Strings(w226, w216) -> (w225:string)
            n131 = local write "midVar_Content"(w225) -> ()
          }
          frame "body_detail_ILD" {
            n132 = for {
              tunnel: string[] ["Port1-Port2: TD-RD", "Port1-Port2: RD-TD"] -> [w248] mode=indexing
              i -> [w236]
              n133 = Increment(x=w236) -> (x+1=w240:i32)
              n134 = Number To Decimal String(number=w240) -> (decimal integer string=w251:string)  [unwired: 1 in]
              n135 = Search and Replace String(input string="            <SubItemTest ID=\"@N@\" name=\"@I@\">\n                <TestResult BoardFlag=\"1\" ID=\"1\" SerialNumber=\"@L@\">\n                    <Outcome value=\"Passed\"/>\n                    <Description>@V@</Description>\n                    <TestData>\n                        <c:Datum xsi:type=\"c:string\">\n                            <c:Value>max value</c:Value>\n                        </c:Datum>\n                     </TestData>\n                </TestResult>\n            </SubItemTest>", search string="@N@" ("搜索字符串"), replace string=w251) -> (result string=w250:string)  [unwired: 5 in, 3 out]
              n136 = local read "input_str_label"() -> (w245:string)
              n137 = Search and Replace String(input string=w250, search string="@I@" ("搜索字符串"), replace string=w248) -> (result string=w247:string)  [unwired: 5 in, 3 out]
              n138 = Search and Replace String(input string=w247, search string="@L@" ("搜索字符串"), replace string=w245) -> (result string=w238:string)  [unwired: 5 in, 3 out]
              n139 = Index Array(array="input_array_ILD_Max", index=w236) -> (element=w242:string)
              n140 = Search and Replace String(input string=w238, search string="@V@" ("搜索字符串"), replace string=w242) -> (result string=w235:string)  [unwired: 5 in, 3 out]
              n141 = local read "midVar_Content"() -> (w244:string)
              n142 = Concatenate Strings(w244, w235) -> (w241:string)
              n143 = local write "midVar_Content"(w241) -> ()
            }
          }
          frame "body_e_ILD" {
            n144 = local read "midVar_Content"() -> (w256:string)
            n145 = Concatenate Strings(w256, "        </ItemTest>") -> (w255:string)
            n146 = local write "midVar_Content"(w255) -> ()
          }
          frame "body_s_Termiantion" {
            n147 = local read "midVar_time"() -> (w262:string[])
            n148 = Index Array(array=w262, index #1=4 ("索引"), index #2=5 ("索引")) -> (element #1=w273:string, element #2=w270:string)
            n149 = Search and Replace String(input string="        <ItemTest ID=\"5\" name=\"Differential Impedance Termination\" startDateTime=\"@T1@\" endDateTime=\"@T2@\">\n            <TestResult BoardFlag=\"1\" ID=\"1\" SerialNumber=\"@L@\" ValueFlag=\"0\">\n                <Outcome value=\"@R@\"/>\n                <Description>NoDesc</Description>\n            </TestResult> ", search string="@T1@" ("搜索字符串"), replace string=w273) -> (result string=w272:string)  [unwired: 5 in, 3 out]
            n150 = Search and Replace String(input string=w272, search string="@T2@" ("搜索字符串"), replace string=w270) -> (result string=w265:string)  [unwired: 5 in, 3 out]
            n151 = local read "input_str_label"() -> (w264:string)
            n152 = Search and Replace String(input string=w265, search string="@L@" ("搜索字符串"), replace string=w264) -> (result string=w260:string)  [unwired: 5 in, 3 out]
            n153 = local read "TDD"() -> (w257:string)
            n154 = local read "midVar_Content"() -> (w269:string)
            n155 = Search and Replace String(input string=w260, search string="@R@" ("搜索字符串"), replace string=w257) -> (result string=w259:string)  [unwired: 5 in, 3 out]
            n156 = Concatenate Strings(w269, w259) -> (w268:string)
            n157 = local write "midVar_Content"(w268) -> ()
          }
          frame "body_detail_Termiantion" {
            n158 = for {
              tunnel: string[] ["Termiantion_TD:ZDD11", "Termiantion_TD:ZDD22", "Termiantion_RD:ZDD11", "Termiantion_RD:ZDD22"] -> [w294] mode=indexing
              i -> [w281]
              n159 = Increment(x=w281) -> (x+1=w283:i32)
              n160 = Number To Decimal String(number=w283) -> (decimal integer string=w297:string)  [unwired: 1 in]
              n161 = Search and Replace String(input string="            <SubItemTest ID=\"@N@\" name=\"@I@\">\n                <TestResult BoardFlag=\"1\" ID=\"1\" SerialNumber=\"@L@\">\n                    <Outcome value=\"Passed\"/>\n                    <Description>@V@</Description>\n                    <TestData>\n                        <c:Datum xsi:type=\"c:string\">\n                            <c:Value>@S@</c:Value>\n                        </c:Datum>\n                     </TestData>\n                </TestResult>\n            </SubItemTest>", search string="@N@" ("搜索字符串"), replace string=w297) -> (result string=w296:string)  [unwired: 5 in, 3 out]
              n162 = local read "input_str_label"() -> (w291:string)
              n163 = Search and Replace String(input string=w296, search string="@I@" ("搜索字符串"), replace string=w294) -> (result string=w293:string)  [unwired: 5 in, 3 out]
              n164 = case shown="2" w281 {
                tunnel: [w302 w305 w308 w311] -> w288
                frame 0, Default {
                  n165 = local read "input_array_TDD11"() -> (w301:string[])
                  n166 = Index Array(array=w301, index=0 ("索引")) -> (element=w302:string)
                }
                frame 1 {
                  n167 = local read "input_array_TDD22"() -> (w304:string[])
                  n168 = Index Array(array=w304, index=0 ("索引")) -> (element=w305:string)
                }
                frame 2 {
                  n169 = local read "input_array_TDD11"() -> (w307:string[])
                  n170 = Index Array(array=w307, index=2 ("索引")) -> (element=w308:string)
                }
                frame 3 {
                  n171 = local read "input_array_TDD22"() -> (w310:string[])
                  n172 = Index Array(array=w310, index=2 ("索引")) -> (element=w311:string)
                }
              }
              n173 = Search and Replace String(input string=w293, search string="@L@" ("搜索字符串"), replace string=w291) -> (result string=w282:string)  [unwired: 5 in, 3 out]
              n174 = local read "input_array_impSpec"() -> (w279:string[])
              n175 = Search and Replace String(input string=w282, search string="@V@" ("搜索字符串"), replace string=w288) -> (result string=w280:string)  [unwired: 5 in, 3 out]
              n176 = local read "midVar_Content"() -> (w290:string)
              n177 = Index Array(array=w279, index=0 ("索引")) -> (element=w278:string)
              n178 = Search and Replace String(input string=w280, search string="@S@" ("搜索字符串"), replace string=w278) -> (result string=w285:string)  [unwired: 5 in, 3 out]
              n179 = Concatenate Strings(w290, w285) -> (w284:string)
              n180 = local write "midVar_Content"(w284) -> ()
            }
          }
          frame "body_e_Termiantion" {
            n181 = local read "midVar_Content"() -> (w315:string)
            n182 = Concatenate Strings(w315, "        </ItemTest>") -> (w314:string)
            n183 = local write "midVar_Content"(w314) -> ()
          }
          frame "body_s_Cable area" {
            n184 = local read "midVar_time"() -> (w321:string[])
            n185 = Index Array(array=w321, index #1=5 ("索引"), index #2=6 ("索引")) -> (element #1=w332:string, element #2=w329:string)
            n186 = Search and Replace String(input string="        <ItemTest ID=\"6\" name=\"Differential Impedance Cable\" startDateTime=\"@T1@\" endDateTime=\"@T2@\">\n            <TestResult BoardFlag=\"1\" ID=\"1\" SerialNumber=\"@L@\" ValueFlag=\"0\">\n                <Outcome value=\"@R@\"/>\n                <Description>NoDesc</Description>\n            </TestResult> ", search string="@T1@" ("搜索字符串"), replace string=w332) -> (result string=w331:string)  [unwired: 5 in, 3 out]
            n187 = Search and Replace String(input string=w331, search string="@T2@" ("搜索字符串"), replace string=w329) -> (result string=w324:string)  [unwired: 5 in, 3 out]
            n188 = local read "input_str_label"() -> (w323:string)
            n189 = Search and Replace String(input string=w324, search string="@L@" ("搜索字符串"), replace string=w323) -> (result string=w319:string)  [unwired: 5 in, 3 out]
            n190 = local read "midVar_Content"() -> (w328:string)
            n191 = local read "TDD"() -> (w316:string)
            n192 = Search and Replace String(input string=w319, search string="@R@" ("搜索字符串"), replace string=w316) -> (result string=w318:string)  [unwired: 5 in, 3 out]
            n193 = Concatenate Strings(w328, w318) -> (w327:string)
            n194 = local write "midVar_Content"(w327) -> ()
          }
          frame "body_detail_Cable area" {
            n195 = for {
              tunnel: string[] ["Cable area_TD:ZDD11", "Cable area_TD:ZDD22", "Cable area_RD:ZDD11", "Cable area_RD:ZDD22"] -> [w353] mode=indexing
              i -> [w342]
              n196 = Increment(x=w342) -> (x+1=w344:i32)
              n197 = Number To Decimal String(number=w344) -> (decimal integer string=w356:string)  [unwired: 1 in]
              n198 = Search and Replace String(input string="            <SubItemTest ID=\"@N@\" name=\"@I@\">\n                <TestResult BoardFlag=\"1\" ID=\"1\" SerialNumber=\"@L@\">\n                    <Outcome value=\"Passed\"/>\n                    <Description>@V@</Description>\n                    <TestData>\n                        <c:Datum xsi:type=\"c:string\">\n                            <c:Value>@S@</c:Value>\n                        </c:Datum>\n                     </TestData>\n                </TestResult>\n            </SubItemTest>", search string="@N@" ("搜索字符串"), replace string=w356) -> (result string=w355:string)  [unwired: 5 in, 3 out]
              n199 = local read "input_str_label"() -> (w350:string)
              n200 = Search and Replace String(input string=w355, search string="@I@" ("搜索字符串"), replace string=w353) -> (result string=w352:string)  [unwired: 5 in, 3 out]
              n201 = case shown="3" w342 {
                tunnel: [w361 w364 w367 w370] -> w341
                frame 0, Default {
                  n202 = local read "input_array_TDD11"() -> (w360:string[])
                  n203 = Index Array(array=w360, index=1 ("索引")) -> (element=w361:string)
                }
                frame 1 {
                  n204 = local read "input_array_TDD22"() -> (w363:string[])
                  n205 = Index Array(array=w363, index=1 ("索引")) -> (element=w364:string)
                }
                frame 2 {
                  n206 = local read "input_array_TDD11"() -> (w366:string[])
                  n207 = Index Array(array=w366, index=3 ("索引")) -> (element=w367:string)
                }
                frame 3 {
                  n208 = local read "input_array_TDD11"() -> (w369:string[])
                  n209 = Index Array(array=w369, index=3 ("索引")) -> (element=w370:string)
                }
              }
              n210 = Search and Replace String(input string=w352, search string="@L@" ("搜索字符串"), replace string=w350) -> (result string=w343:string)  [unwired: 5 in, 3 out]
              n211 = Search and Replace String(input string=w343, search string="@V@" ("搜索字符串"), replace string=w341) -> (result string=w340:string)  [unwired: 5 in, 3 out]
              n212 = local read "input_array_impSpec"() -> (w338:string[])
              n213 = local read "midVar_Content"() -> (w349:string)
              n214 = Index Array(array=w338, index=1 ("索引")) -> (element=w337:string)
              n215 = Search and Replace String(input string=w340, search string="@S@" ("搜索字符串"), replace string=w337) -> (result string=w346:string)  [unwired: 5 in, 3 out]
              n216 = Concatenate Strings(w349, w346) -> (w345:string)
              n217 = local write "midVar_Content"(w345) -> ()
            }
          }
          frame "body_e_Cable area" {
            n218 = local read "midVar_Content"() -> (w374:string)
            n219 = Concatenate Strings(w374, "        </ItemTest>") -> (w373:string)
            n220 = local write "midVar_Content"(w373) -> ()
          }
          frame "body_s_Next" {
            n221 = local read "midVar_time"() -> (w380:string[])
            n222 = Index Array(array=w380, index #1=6 ("索引"), index #2=7 ("索引")) -> (element #1=w391:string, element #2=w388:string)
            n223 = Search and Replace String(input string="        <ItemTest ID=\"7\" name=\"Next\" startDateTime=\"@T1@\" endDateTime=\"@T2@\">\n            <TestResult BoardFlag=\"1\" ID=\"1\" SerialNumber=\"@L@\" ValueFlag=\"0\">\n                <Outcome value=\"@R@\"/>\n                <Description>NoDesc</Description>\n            </TestResult> ", search string="@T1@" ("搜索字符串"), replace string=w391) -> (result string=w390:string)  [unwired: 5 in, 3 out]
            n224 = Search and Replace String(input string=w390, search string="@T2@" ("搜索字符串"), replace string=w388) -> (result string=w383:string)  [unwired: 5 in, 3 out]
            n225 = local read "input_str_label"() -> (w382:string)
            n226 = Search and Replace String(input string=w383, search string="@L@" ("搜索字符串"), replace string=w382) -> (result string=w378:string)  [unwired: 5 in, 3 out]
            n227 = local read "NEXT"() -> (w375:string)
            n228 = local read "midVar_Content"() -> (w387:string)
            n229 = Search and Replace String(input string=w378, search string="@R@" ("搜索字符串"), replace string=w375) -> (result string=w377:string)  [unwired: 5 in, 3 out]
            n230 = Concatenate Strings(w387, w377) -> (w386:string)
            n231 = local write "midVar_Content"(w386) -> ()
          }
          frame "body_detail_Next" {
            n232 = for {
              tunnel: string[] ["Next_TX-RX", "Next_RX-TX"] -> [w408] mode=indexing
              i -> [w397]
              n233 = Increment(x=w397) -> (x+1=w400:i32)
              n234 = Number To Decimal String(number=w400) -> (decimal integer string=w411:string)  [unwired: 1 in]
              n235 = Search and Replace String(input string="            <SubItemTest ID=\"@N@\" name=\"@I@\">\n                <TestResult BoardFlag=\"1\" ID=\"1\" SerialNumber=\"@L@\">\n                    <Outcome value=\"Passed\"/>\n                    <Description>@V@</Description>\n                    <TestData>\n                        <c:Datum xsi:type=\"c:string\">\n                            <c:Value>5000MHZ</c:Value>\n                        </c:Datum>\n                     </TestData>\n                </TestResult>\n            </SubItemTest>", search string="@N@" ("搜索字符串"), replace string=w411) -> (result string=w410:string)  [unwired: 5 in, 3 out]
              n236 = local read "input_str_label"() -> (w405:string)
              n237 = Search and Replace String(input string=w410, search string="@I@" ("搜索字符串"), replace string=w408) -> (result string=w407:string)  [unwired: 5 in, 3 out]
              n238 = Search and Replace String(input string=w407, search string="@L@" ("搜索字符串"), replace string=w405) -> (result string=w399:string)  [unwired: 5 in, 3 out]
              n239 = Index Array(array="input_array_Next", index=w397) -> (element=w402:string)
              n240 = Search and Replace String(input string=w399, search string="@V@" ("搜索字符串"), replace string=w402) -> (result string=w396:string)  [unwired: 5 in, 3 out]
              n241 = local read "midVar_Content"() -> (w404:string)
              n242 = Concatenate Strings(w404, w396) -> (w401:string)
              n243 = local write "midVar_Content"(w401) -> ()
            }
          }
          frame "body_e_Next" {
            n244 = local read "midVar_Content"() -> (w417:string)
            n245 = Concatenate Strings(w417, "        </ItemTest>") -> (w416:string)
            n246 = local write "midVar_Content"(w416) -> ()
          }
          frame "tail" {
            # "</ResultSet>\n    <TestProgram Productline=\"XT-113\" Product=\"SFP+\">\n        <c:Definition name=\"HPTS\" version=\"6.0\">\n            <c:Description>NoDesc</c:Description> \n        </c:Definition>\n    </TestProgram>\n    <!--  ATE--> \n    <TestStation AteName=\"TDR\" AteVersion=\"1.001\" /> \n    <!--  SerialNumber--> \n    <UUT UutType=\"hardware\">\n        <SerialNumber>@L@</SerialNumber> \n        <ItemName>SFP+</ItemName>\n        <ItemCode>@C@</ItemCode> \n    </UUT>\n    <WorkOrder>\n        <WorkItem name=\"a\">\n            <c:Datum xsi:type=\"c:string\">\n                <c:Value>SPZS06311C1</c:Value> \n            </c:Datum>\n        </WorkItem>\n    </WorkOrder>\n</TestResults"
            n247 = Concatenate Strings("\"" ("字符串"), "FileVer", "\"" ("字符串")) -> (w422:string)
            n248 = local read "input_str_product"() -> (w444:string)
            n249 = Search and Replace String(input string="    </ResultSet>\n    <TestProgram Productline=\"XT-113\" Product=\"SFP+\">\n        <c:Definition name=\"VNA\" version=@Ver@>\n            <c:Description>@Path@</c:Description> \n        </c:Definition>\n    </TestProgram>\n    <!--  ATE--> \n    <TestStation AteName=@PCName@ AteVersion=\"1.001\" /> \n    <!--  SerialNumber--> \n    <UUT UutType=\"hardware\">\n        <SerialNumber>@L@</SerialNumber> \n        <ItemName>SFP+</ItemName>\n        <ItemCode>@C@</ItemCode> \n    </UUT>\n    <WorkOrder>\n        <WorkItem name=\"a\">\n            <c:Datum xsi:type=\"c:string\">\n                <c:Value>SPZS06311C1</c:Value> \n            </c:Datum>\n        </WorkItem>\n    </WorkOrder>\n</TestResults>", search string="@Ver@" ("搜索字符串"), replace string=w422) -> (result string=w431:string)  [unwired: 5 in, 3 out]
            n250 = call "PCsName.vi"() -> ("Computer Name"=w421:string)
            n251 = Search and Replace String(input string=w431, search string="@Path@" ("搜索字符串"), replace string="FilePath") -> (result string=w429:string)  [unwired: 5 in, 3 out]
            n252 = local read "input_str_label"() -> (w441:string)
            n253 = Concatenate Strings("\"" ("字符串"), w421, "\"" ("字符串")) -> (w418:string)
            n254 = Search and Replace String(input string=w429, search string="@PCName@" ("搜索字符串"), replace string=w418) -> (result string=w427:string)  [unwired: 5 in, 3 out]
            n255 = Search and Replace String(input string=w427, search string="@P@" ("搜索字符串"), replace string=w444) -> (result string=w443:string)  [unwired: 5 in, 3 out]
            n256 = Search and Replace String(input string=w443, search string="@L@" ("搜索字符串"), replace string=w441) -> (result string=w436:string)  [unwired: 5 in, 3 out]
            n257 = local read "input_str_CustomerPN"() -> (w434:string)
            n258 = local read "midVar_Content"() -> (w440:string)
            n259 = Search and Replace String(input string=w436, search string="@C@" ("搜索字符串"), replace string=w434) -> (result string=w437:string)  [unwired: 5 in, 3 out]
            n260 = Concatenate Strings(w440, w437) -> (w439:string)
            n261 = local write "midVar_Content"(w439) -> ()
          }
          frame "end" {
            n262 = local read "midVar_Content"() -> (w448:string)
            n263 = Open/Create/Replace File(file path (use dialog)="路径", operation (0:open)=T1."open or create" ("操作(0:open)")) -> (refnum out=w450:refnum<file>)  [unwired: 4 in, 2 out]
            n264 = Write to Text File(file (use dialog)=w450, text=w448) -> (refnum out=w449:refnum<file>)  [unwired: 2 in, 2 out]
            n265 = Close File(refnum=w449) -> ()  [unwired: 1 in, 2 out]
          }
        }
        n266 = local write "midVar_state"(w55) -> ()
      }
    }
  }
